vi "Send Test_Name.vi"(8 "error in":errorcluster, 10 "Test Name":string, 11 "Engine in":refnum<class "Engine.lvclass">) -> (0 "error out":errorcluster, 3 "Engine out":refnum<class "Engine.lvclass">)   [LabVIEW 2023, in "Engine.lvlib" / "Engine.lvclass"]
doc: "Trigger the Update Test Name Event (allowing components to update any references to the Test name).\n\nThen enqueue a close and open operation to the report generator. (ensuring reports are generated with association to the name of the test)"
uses:
  Project/Engine.lvclass
  Project/Engine.lvclass/Engine.ctl
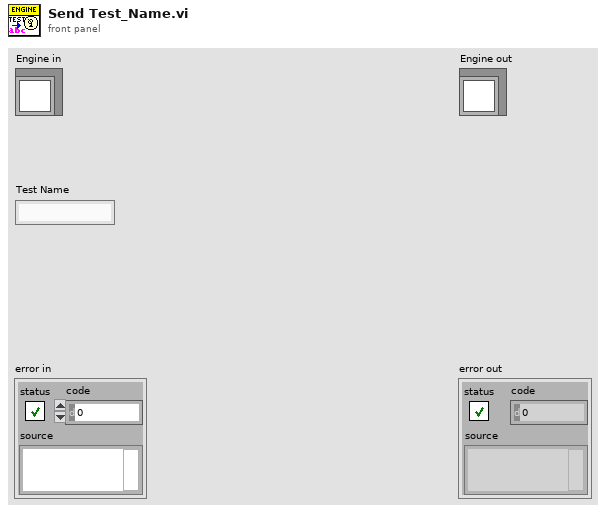
[diagram p1: front panel]
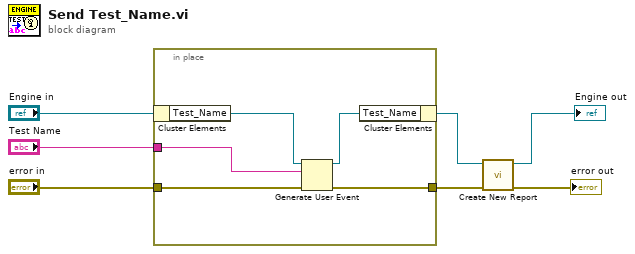
[diagram p0: block diagram]
diagram:
  n1 = in-place {
    in-place-border: "error in" -> [w10]
    in-place-border: [w9] -> w2
    in-place-border: "Test Name" -> [w8]
    n2 = in-place-cluster #1("Engine in") -> ("Test_Name"=w12:refnum<user-event>)
    n3 = Generate User Event(user event=w12, event data cluster=w8, error in=w10) -> (user event out=w11:refnum<user-event>, error out=w9:errorcluster)  [unwired: 1 in]
    n4 = in-place-cluster #1("Test_Name"=w11) -> (w4:refnum<class "Engine.lvclass">)
  }
  n5 = call "Create New Report.vi"("error in"=w2, "Engine in"=w4) -> ("error out"=→"error out":errorcluster, "Engine out"=→"Engine out":refnum<class "Engine.lvclass">)  [unwired: 8 in]
